vi "gwyscan create path octave 2d.vi"(0 "xypos":dbl[](array[numeric]), 1 "yreal":dbl, 2 "yoffset":dbl, 5 "order":i32, 7 "noctaves":i32, 9 "xreal":dbl, 11 "error in (no error)":errorcluster, 12 "xoffset":dbl) -> (4 "xypos out":dbl[](array[numeric]), 6 "function return":i32, 15 "error out":errorcluster)   [LabVIEW 2016, in "libgwyscan.lvlib"]
doc: "GWYSCANDLL_API int gwyscan_create_path_octave_2d(double *xypos, int order, int noctaves, double xreal, double yreal, double xoffset, double yoffset);"
uses:
  libgwyscan.lvlib
  libgwyscan.dll
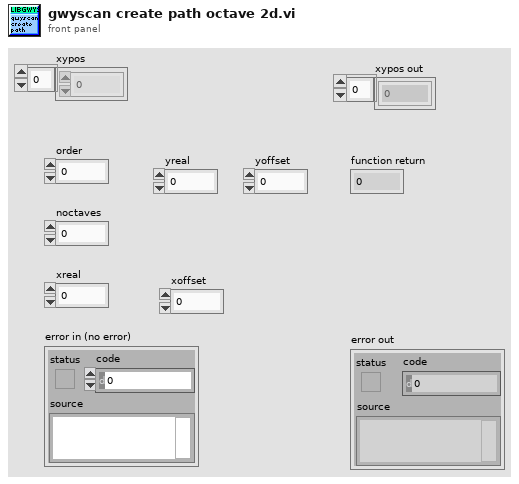
[diagram p1: front panel]
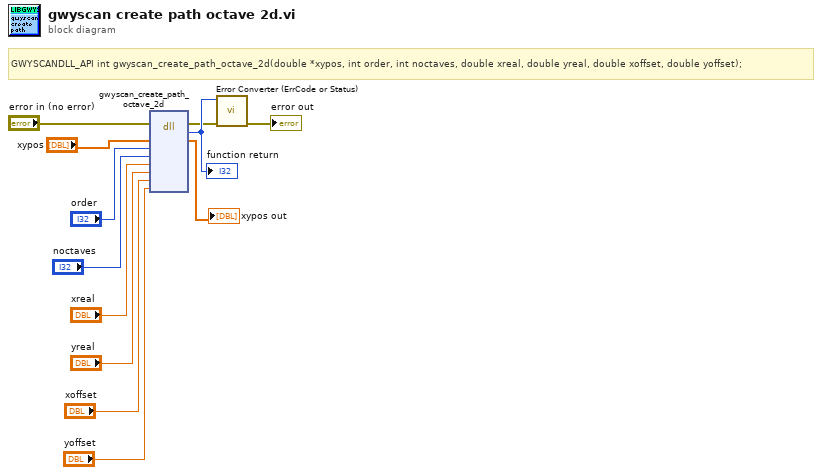
[diagram p0: block diagram]
diagram:
  # "GWYSCANDLL_API int gwyscan_create_path_octave_2d(double *xypos, int order, int noctaves, double xreal, double yreal, double xoffset, double yoffset);"
  n1 = dll-call lib="PTH2abs CUsersCharlÃ¨ne BrillardDesktoplbni-lbniAFMController-BetaVersionv2.0.16-20190611 libgwyscan-1.2-labview2015-win32libgwyscan.*" fn="gwyscan_create_path_octave_2d"(error in="error in (no error)", "xypos"="xypos", "order"="order", "noctaves"="noctaves", "xreal"="xreal", "yreal"="yreal", "xoffset"="xoffset", "yoffset"="yoffset") -> (error out=w3:errorcluster, "return type"=w12:i32, "xypos"=→"xypos out":dbl[])  [unwired: 8 in, 1 out]
  "function return" <- w12
  n2 = call "Error Converter (ErrCode or Status).vi"("error in (no error)"=w3, "error code"=w12) -> ("error out"=→"error out":errorcluster)  [unwired: 9 in]
